vi "DUT Write.vi"(0 "Digital TSM In":T2, 5 "Per Site Data In":u8[](array[numeric]), 11 "error in (no error)":errorcluster, 13 "Operation":T1) -> (4 "Digital TSM Out":T2, 6 "Per-Site Pass":bool[](array[boolean]), 8 "Per Site Data Out":u8[](array[numeric]), 15 "error out":errorcluster)   [LabVIEW 2020]
uses:
  Instrument Control/Digital/TSM/TSM SSC Digital.ctl
  <vilib>/NI_TestStand_SemiconductorModule/NI_TestStand_Semiconductor_Module.lvlibp/PinMap/Digital Pattern/PinQueryContext/DigitalPatternPinQueryContext.lvclass
  Instrument Control/Digital/SSC Digital/SSC Digital.ctl
  Typedefs/DUT Write Commands.ctl
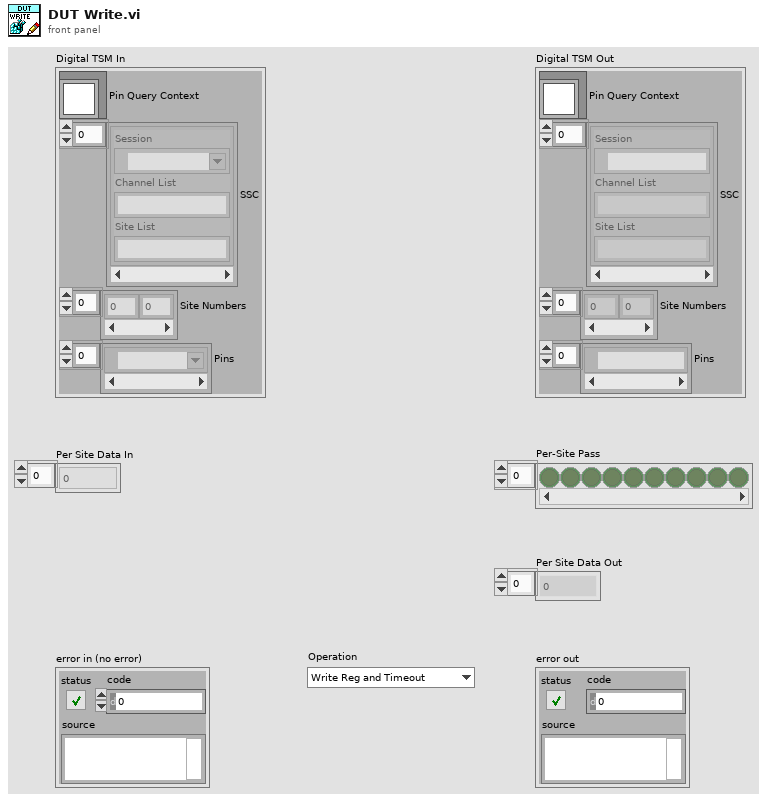
[diagram p1: front panel]
types:
  T1 = typedef "DUT Write Commands.ctl" = enum16{"Write Reg and Timeout", "Write Reg and Nmode Cmd", "Program OTP"}
  T2 = typedef "TSM SSC Digital.ctl" = cluster{"Pin Query Context":refnum<class "DigitalPatternPinQueryContext.lvclass">, "SSC":T3[], "Site Numbers":i32[], "Pins":tag[]}
  T3 = typedef "SSC Digital.ctl" = cluster{"Session":refnum<k15>, "Channel List":string, "Site List":string}
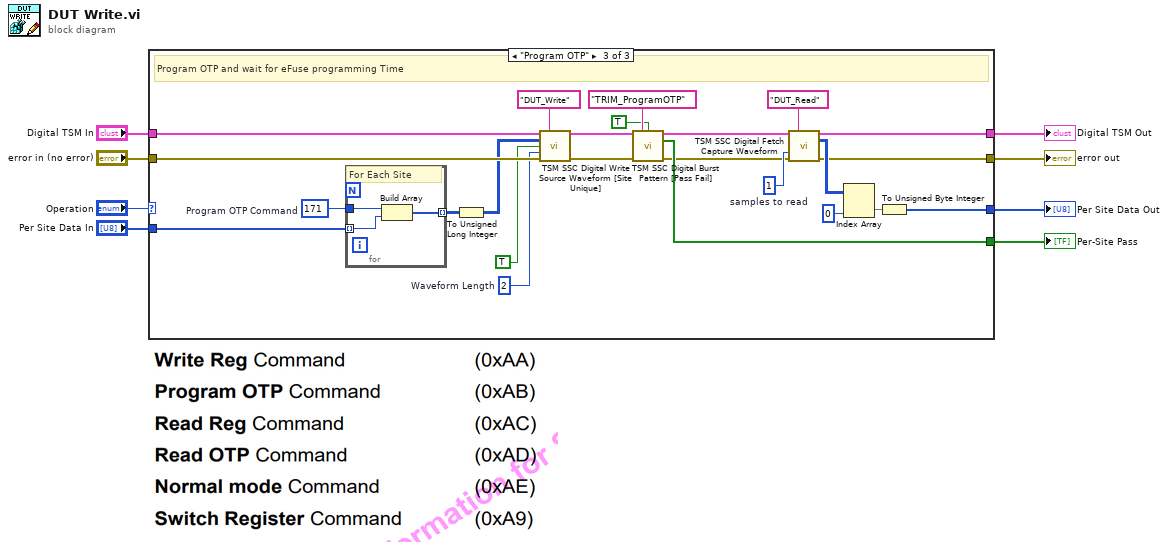
[diagram p0: block diagram]
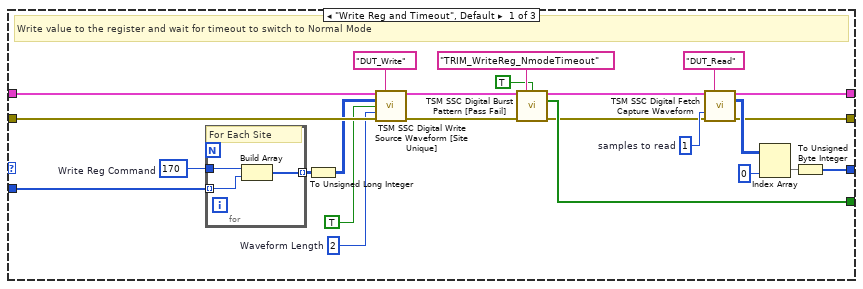
[diagram p2: hidden frame]
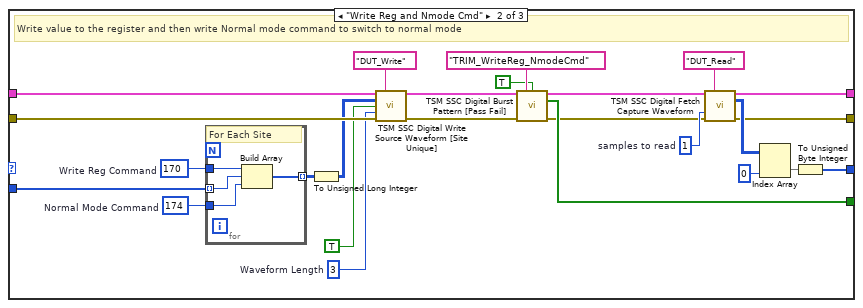
[diagram p3: hidden frame]
diagram:
  n1 = case shown="\"Program OTP\"" "Operation" {
    tunnel: "Digital TSM In" -> [w31 w59 w87]
    tunnel: "error in (no error)" -> [w30 w58 w86]
    tunnel: "Per Site Data In" -> [w29 w57 w85]
    tunnel: [w22 w50 w78] -> w5
    tunnel: [w16 w44 w72] -> w4
    tunnel: [w12 w40 w68] -> w3
    tunnel: [w11 w39 w67] -> w2
    frame "Write Reg and Timeout", Default {
      w9 = u8 170  # Write Reg Command
      w21 = 1  # samples to read
      w27 = 2  # Waveform Length
      # "Write value to the register and wait for timeout to switch to Normal Mode"
      n2 = for {
        tunnel: w29 -> [w34] mode=indexing
        tunnel: w9 -> [w35]
        tunnel: [w33] -> w28 mode=indexing
        # "For Each Site"
        n3 = Build Array(w35, w34) -> (w33:u8[])
      }
      n4 = To Unsigned Long Integer(number=w28) -> (unsigned 32bit integer=w10:u32[][])
      n5 = call "TSM SSC Digital Write Source Waveform [Site Unique].vi"("Digital - Sessions in"=w31, "Waveform Name"="DUT_Write", "Per-Site Waveforms"=w10, "Expand to Minimum Size?"=TRUE, "Minimum Size"=w27, "error in"=w30) -> ("Digital - Sessions out"=w24:T2, "error out"=w25:errorcluster)  [unwired: 8 in]
      n6 = call "TSM SSC Digital Burst Pattern [Pass Fail].vi"("Digital TSM In"=w24, "Start Label"="TRIM_WriteReg_NmodeTimeout", "select digital function?"=TRUE, "error in"=w25) -> ("Digital TSM out"=w13:T2, "Per-Site Pass"=w22:bool[], "error out"=w14:errorcluster)  [unwired: 9 in]
      n7 = call "TSM SSC Digital Fetch Capture Waveform.vi"("Digital TSM In"=w13, "Waveform Name"="DUT_Read", "samples to read"=w21, "error in"=w14) -> ("Digital TSM Out"=w12:T2, "Per-Site Waveforms"=w19:u32[][], "error out"=w11:errorcluster)  [unwired: 9 in]
      n8 = Index Array(array=w19, index (col)=0 ("disabled index (col)")) -> (element=w17:u32[])  [unwired: 1 in]
      n9 = To Unsigned Byte Integer(number=w17) -> (unsigned 8bit integer=w16:u8[])
    }
    frame "Write Reg and Nmode Cmd" {
      w36 = u8 174  # Normal Mode Command
      w37 = u8 170  # Write Reg Command
      w49 = 1  # samples to read
      w55 = 3  # Waveform Length
      # "Write value to the register and then write Normal mode command to switch to normal mode"
      n10 = for {
        tunnel: w57 -> [w63] mode=indexing
        tunnel: w37 -> [w64]
        tunnel: [w62] -> w56 mode=indexing
        tunnel: w36 -> [w61]
        # "For Each Site"
        n11 = Build Array(w64, w63, w61) -> (w62:u8[])
      }
      n12 = To Unsigned Long Integer(number=w56) -> (unsigned 32bit integer=w38:u32[][])
      n13 = call "TSM SSC Digital Write Source Waveform [Site Unique].vi"("Digital - Sessions in"=w59, "Waveform Name"="DUT_Write", "Per-Site Waveforms"=w38, "Expand to Minimum Size?"=TRUE, "Minimum Size"=w55, "error in"=w58) -> ("Digital - Sessions out"=w52:T2, "error out"=w53:errorcluster)  [unwired: 8 in]
      n14 = call "TSM SSC Digital Burst Pattern [Pass Fail].vi"("Digital TSM In"=w52, "Start Label"="TRIM_WriteReg_NmodeCmd", "select digital function?"=TRUE, "error in"=w53) -> ("Digital TSM out"=w41:T2, "Per-Site Pass"=w50:bool[], "error out"=w42:errorcluster)  [unwired: 9 in]
      n15 = call "TSM SSC Digital Fetch Capture Waveform.vi"("Digital TSM In"=w41, "Waveform Name"="DUT_Read", "samples to read"=w49, "error in"=w42) -> ("Digital TSM Out"=w40:T2, "Per-Site Waveforms"=w47:u32[][], "error out"=w39:errorcluster)  [unwired: 9 in]
      n16 = Index Array(array=w47, index (col)=0 ("disabled index (col)")) -> (element=w45:u32[])  [unwired: 1 in]
      n17 = To Unsigned Byte Integer(number=w45) -> (unsigned 8bit integer=w44:u8[])
    }
    frame "Program OTP" {
      w65 = u8 171  # Program OTP Command
      w77 = 1  # samples to read
      w83 = 2  # Waveform Length
      # "Program OTP and wait for eFuse programming Time"
      n18 = for {
        tunnel: w85 -> [w90] mode=indexing
        tunnel: w65 -> [w91]
        tunnel: [w89] -> w84 mode=indexing
        # "For Each Site"
        n19 = Build Array(w91, w90) -> (w89:u8[])
      }
      n20 = To Unsigned Long Integer(number=w84) -> (unsigned 32bit integer=w66:u32[][])
      n21 = call "TSM SSC Digital Write Source Waveform [Site Unique].vi"("Digital - Sessions in"=w87, "Waveform Name"="DUT_Write", "Per-Site Waveforms"=w66, "Expand to Minimum Size?"=TRUE, "Minimum Size"=w83, "error in"=w86) -> ("Digital - Sessions out"=w80:T2, "error out"=w81:errorcluster)  [unwired: 8 in]
      n22 = call "TSM SSC Digital Burst Pattern [Pass Fail].vi"("Digital TSM In"=w80, "Start Label"="TRIM_ProgramOTP", "select digital function?"=TRUE, "error in"=w81) -> ("Digital TSM out"=w69:T2, "Per-Site Pass"=w78:bool[], "error out"=w70:errorcluster)  [unwired: 9 in]
      n23 = call "TSM SSC Digital Fetch Capture Waveform.vi"("Digital TSM In"=w69, "Waveform Name"="DUT_Read", "samples to read"=w77, "error in"=w70) -> ("Digital TSM Out"=w68:T2, "Per-Site Waveforms"=w75:u32[][], "error out"=w67:errorcluster)  [unwired: 9 in]
      n24 = Index Array(array=w75, index (col)=0 ("disabled index (col)")) -> (element=w73:u32[])  [unwired: 1 in]
      n25 = To Unsigned Byte Integer(number=w73) -> (unsigned 8bit integer=w72:u8[])
    }
  }
  "error out" <- w2
  "Digital TSM Out" <- w3
  "Per-Site Pass" <- w5
  "Per Site Data Out" <- w4
